vi "SetGetStatMeasParams.vi"() -> ()   [LabVIEW 2017]
uses:
  AT901 API/Structures/Struct StationaryModeData.ctl
panel:
  out "StationaryModeParams":T1={"Use ADM"=TRUE, "lMeasTime"=0}
  in  "StationaryModeData":T1={"Use ADM"=TRUE, "lMeasTime"=0}
  out "error out":errorcluster
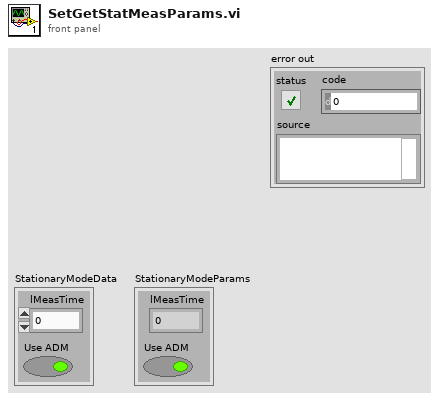
[diagram p1: front panel]
types:
  T1 = typedef "Struct StationaryModeData.ctl" = cluster{"Use ADM":bool, "lMeasTime":i32}
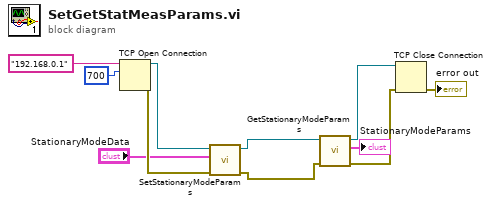
[diagram p0: block diagram]
diagram:
  n1 = TCP Open Connection(address="192.168.0.1", remote port or service name=u16 700) -> (connection ID=w8:refnum<k5>, error out=w3:errorcluster)  [unwired: 3 in]
  n2 = call "SetStationaryModeParams.vi"("error in (no error)"=w3, "StationaryModeData"="StationaryModeData", "TCP Network Connection in"=w8) -> ("error out"=w4:errorcluster, "TCP Network Connection out"=w7:refnum<k5>)  [unwired: 5 in, 2 out]
  n3 = call "GetStationaryModeParams.vi"("error in (no error)"=w4, "TCP Network Connection in"=w7) -> ("error out"=w5:errorcluster, "StationaryModeParams"=→"StationaryModeParams":T1, "TCP Network Connection out"=w6:refnum<k5>)  [unwired: 5 in, 2 out]
  n4 = TCP Close Connection(connection ID=w6, error in (no error)=w5) -> (error out=→"error out":errorcluster)  [unwired: 1 in, 1 out]
